vi "Joystick.vi"(8 "error in (no error)":errorcluster, 10 "Joystick":bool, 11 "Gantry in":refnum<class "A3200.lvclass">) -> (0 "error out":errorcluster, 3 "Gantry out":refnum<class "A3200.lvclass">)   [LabVIEW 2016, in "A3200.lvclass"]
uses:
  A3200.lvclass
  A3200.lvclass/A3200.ctl
  Drivers/Aerotech A3200/Aerotech VIs.lvlib
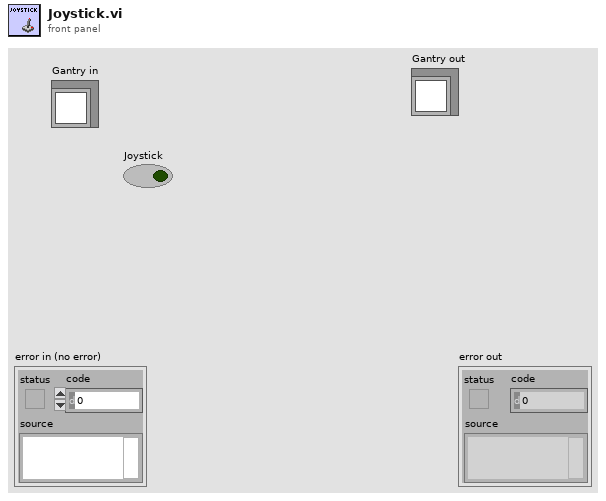
[diagram p1: front panel]
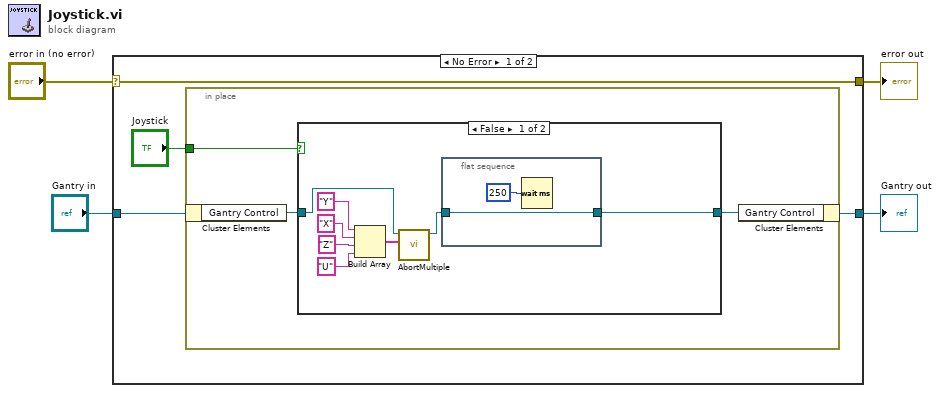
[diagram p0: block diagram]
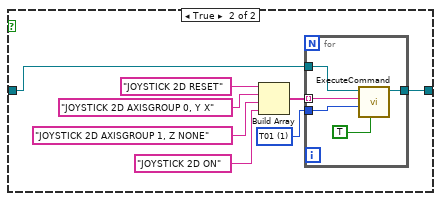
[diagram p2: hidden frame]
diagram:
  n1 = case shown="No Error" "error in (no error)" {
    selector: "error in (no error)" -> [w8 w36]
    tunnel: [w8 w36] -> w3
    tunnel: [w5 w35] -> w1
    tunnel: "Gantry in" -> [w6 w35]
    frame No Error {
      n2 = in-place {
        in-place-border: "Joystick" -> [w11]
        n3 = in-place-cluster #1(w6) -> ("Gantry Control"=w10:refnum<k24>)
        n4 = case shown="False" w11 {
          tunnel: w10 -> [w14 w23]
          tunnel: [w12 w22] -> w9
          frame False {
            n5 = Build Array("Y" ("axis name"), "X", "Z", "U") -> (w15:string[])
            n6 = call "AbortMultiple.vi"("axis names"=w15, "controller in"=w14) -> ("controller out"=w13:refnum<k24>)  [unwired: 8 in, 1 out]
            n7 = flat-sequence {
              tunnel: w13 -> [w21]
              tunnel: [w21] -> w12
              frame #0 {
                n8 = Wait (ms)(milliseconds to wait=u32 250) -> ()  [unwired: 1 out]
              }
            }
          }
          frame True {
            w25 = 1 items=["TLibrary", "T01", "T02", "T03", "T04", "T05", "T06", "T07", "T08", "T09", "T10", "T11", "T12", "T13", "T14", "T15", "T16", "T17", "T18", "T19", "T20", "T21", "T22", "T23", "T24", "T25", "T26", "T27", "T28", "T29", "T30", "T31"] ("taskId")
            n9 = Build Array("JOYSTICK 2D RESET", "JOYSTICK 2D AXISGROUP 0, Y X", "JOYSTICK 2D AXISGROUP 1, Z NONE", "JOYSTICK 2D ON") -> (w26:string[])
            n10 = for {
              tunnel: w26 -> [w34] mode=indexing
              tunnel: w25 -> [w33]
              tunnel: w23 -> [w31]
              tunnel: [w32] -> w22
              n11 = call "ExecuteCommand.vi"("return immediately"=TRUE, "taskId"=w33, "Command Code"=w34, "controller in"=w31) -> ("controller out"=w32:refnum<k24>)  [unwired: 5 in, 2 out]
            }
          }
        }
        n12 = in-place-cluster #1("Gantry Control"=w9) -> (w5:refnum<class "A3200.lvclass">)
      }
    }
    frame Error {
    }
  }
  "error out" <- w3
  "Gantry out" <- w1
